vi "Get SLSC Relay Info.vi"(8 "error in (no error)":errorcluster, 10 "relay index":i32, 11 "SLSC Switch in":refnum<class "SLSC Switch.lvclass">) -> (0 "error out":errorcluster, 2 "SLSC Switch Info":T1, 3 "SLSC Switch out":refnum<class "SLSC Switch.lvclass">)   [LabVIEW 2015, in "SLSC Switch.lvclass"]
uses:
  SLSC Switch.lvclass
  Controls/SLSC Relay Info.ctl
  SLSC Switch.lvclass/SLSC Switch.ctl
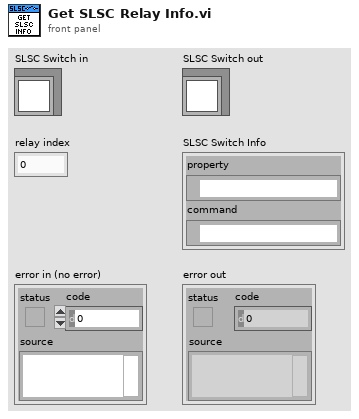
[diagram p1: front panel]
types:
  T1 = typedef "SLSC Switch.lvclass/SLSC Relay Info.ctl" = cluster{"property":refnum<k21>, "command":refnum<k21>}
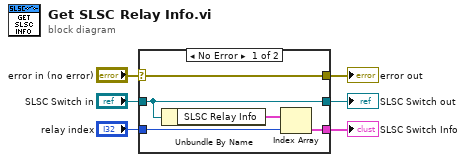
[diagram p0: block diagram]
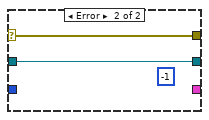
[diagram p2: hidden frame]
diagram:
  n1 = case shown="No Error" "error in (no error)" {
    selector: "error in (no error)" -> [w10 w13]
    tunnel: [w10 w13] -> w5
    tunnel: [w11 w12] -> w3
    tunnel: "SLSC Switch in" -> [w11 w12]
    tunnel: "relay index" -> [w8 _]
    tunnel: [w7 _] -> w1
    frame No Error {
      n2 = Unbundle By Name(w11) -> ("SLSC Relay Info"=w9:T1[])
      n3 = Index Array(array=w9, index=w8) -> (element=w7:T1)
    }
    frame Error {
      (unwired) -1 ("f")
    }
  }
  "error out" <- w5
  "SLSC Switch out" <- w3
  "SLSC Switch Info" <- w1
